vi "Listbox - Route Specification to Connected Routes.vi"(8 "error in (no error)":errorcluster, 10 "route specification":string, 11 "listbox reference":refnum<vi>) -> (0 "error out":errorcluster, 3 "listbox reference out":refnum<vi>)   [LabVIEW 2023, in "SwitchExecController.lvlib"]
uses:
  SwitchExecController.lvlib
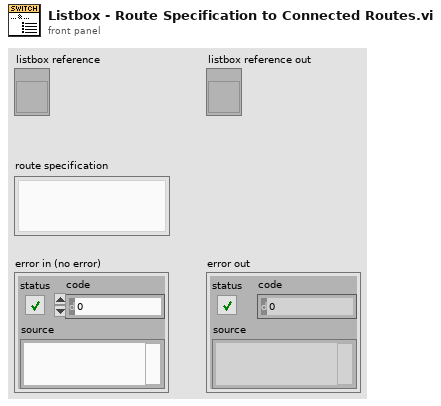
[diagram p1: front panel]
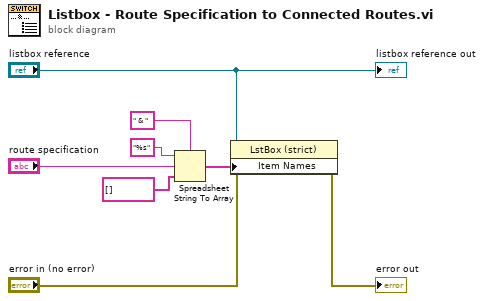
[diagram p0: block diagram]
diagram:
  n1 = Spreadsheet String To Array(delimiter (Tab)=" & ", format string="%s", spreadsheet string="route specification", array type (2D Dbl)=string[] []) -> (array=w1:string[])
  n2 = property class="LstBox (strict)"(reference="listbox reference", error in="error in (no error)", "Item Names"=w1) -> (error out=→"error out":errorcluster)  [unwired: 1 out]
  "listbox reference out" <- "listbox reference"
